vi "Controller with Indicators.vi"() -> ()   [LabVIEW 2009]
doc: "This example shows how to use Simulation Module and Control Design Toolkit together and how to transfer the controller from Design to Simulation. It also uses the 3D Picture Control Toolkit to animate the system.\nThis example is derived from the Quanser (www.quanser.com) 3 DOF Helicopter academic experiment."
uses:
  <vilib>/Simulation/Scripting/Companion Diagram/SimConfigNode/SimDog.xnode
  <vilib>/Simulation/Utility/SIMX SimTime/SIMX SimTime.xnode
  <vilib>/Simulation/SignalArithmetic/SIMX Gain/SIMX Gain.xnode
  <vilib>/Simulation/Implementation/XNodeFramework/AbstractNodes/SimX_SubsystemNode/SimX_SubsystemNode.xnode
  <vilib>/Simulation/Utility/SIMX Halt/SIMX Halt.xnode
  Heli SubVIs/cdex_unwrap signal.vi
  <vilib>/Simulation/SignalArithmetic/Implementation/NILVSim Gain.llb/SIM Gain (scalar).vi
  <vilib>/Simulation/Implementation/Shared/SIMSCR Execution Mode.ctl
  <vilib>/Simulation/Scripting/Companion Diagram/SimConfigNode/_simSolvers.ctl
  <vilib>/Simulation/Scripting/Companion Diagram/SimConfigNode/SimParams.ctl
  <vilib>/Simulation/Utility/Implementation/SIM Time.vi
  <vilib>/Simulation/Utility/Implementation/SIM Halt.vi
  NiRioSrv.dll
  <vilib>/Utility/error.llb/Error Cluster From Error Code.vi
  <vilib>/rvi/errors/niLvFpgaWhatHappensToTopLevelVI.ctl
  <vilib>/rvi/interface/common/niFpgaNodeNameForErrorReporting.ctl
  <vilib>/rvi/errors/niLvFpgaAdjustHostInterfaceError.vi
  <vilib>/rvi/interface/nirviReadWriteControl/nirviReadWriteControl.xnode
  FPGA Bitfiles/sbRIOController.lv~4B_sbRIO-9631_FPGA Main.vi.lvbitx
  <vilib>/userDefined/High Color/nirio_resource_hc.ctl
  <vilib>/rvi/interface/nirviOpenFPGA/nirviOpenFPGA.xnode
  RT/Set to PWM.vi
  <vilib>/rvi/interface/nirviCloseFPGA/nirviCloseFPGA.xnode
  Heli SubVIs/cdex_Position PID.vi
  Heli SubVIs/cdex_Elevation PID.vi
  Heli SubVIs/cdex_Pitch PID.vi
  FPGA/FPGA Main.vi
  RT/Read Encoder Data.vi
  RT/MyGlobal.vi
  <vilib>/Simulation/Implementation/Shared/SIM Bundle Sim Info.vi
  <vilib>/Simulation/Implementation/Shared/SIM Unbundle Sim Info.vi
  <vilib>/Platform/TimedLoop/XDataNode/wakeup.ctl
  <vilib>/Platform/TimedLoop/XDataNode/XDNodeRunTimeDep.lvlib
  <vilib>/Platform/TimedLoop/XDataNode/nitl_modes.ctl
  <vilib>/Platform/TimedLoop/XDataNode/timing_clust.ctl
  <vilib>/Platform/TimedLoop/XDataNode/XDataNode.xnode
  <vilib>/Simulation/Implementation/Shared/NILVSim_Initialize.vi
  <vilib>/Simulation/Implementation/Shared/NILVSim_FinishedLate.vi
  <vilib>/Simulation/Implementation/Shared/NILVSim_Manager.vi
  <vilib>/Simulation/Implementation/Shared/NILVSim_FinalizeModel.vi
  <vilib>/Simulation/Implementation/Shared/NILVSim_GetModelError.vi
  <vilib>/Platform/TimedLoop/XDataNode/loadlvalarms.vi
  <vilib>/Simulation/Implementation/Shared/SIM Fire Discrete SubVI.vi
  <vilib>/Simulation/Scripting/Editor Utilities/SIM subVI execution type.ctl
  <vilib>/Simulation/Scripting/Editor Utilities/SIM subVI tag data.ctl
  <vilib>/FPGAPlugInAG/sbRIO-9631/nirviIntfOpen_sbRIO-9631.vi
  FPGA/FPGA Main NoStartEnc.vi
  FPGA Bitfiles/sbRIOController.lv~4B_sbRIO-9631_FPGA Main NoStartE~C3.lvbitx
  <vilib>/FPGAPlugInAG/sbRIO-9631/nirviIntfClose_sbRIO-9631.vi
panel:
  in  "stop":bool
  out "error out":errorcluster
  in  "GO":bool
  in  "Clock Divider (ticks)":u16=1
  in  "PWM Period (ticks)":u32=100000
  out "Simulation Time":dbl=55.800000000000004 format="%<%H:%M:%S%1u>t"
  out "Measured Pitch Angle":dbl=0.00018032364824244914
  out "Measure Angle":dbl=14.22166948358761
  out "Measured Elevation":dbl=14.497088945408226
  in  "Position Angle Setpoint":dbl(knob) scale=-180.0..180.0
  in  "Elevation Setpoint":dbl(slide) scale=0.0..20.0 scale format="%.2f"
  out "Control Effort [Vf,Vb]":cluster{dbl, dbl}(graph)={-0.0027402268665562613, -0.002740193984032141}
  out "Travel Angle":cluster{"travel position":dbl, "signal out":dbl}(graph)={"travel position"=14.222946670967534, "signal out"=14.22166948358761}
  out "Elevation Angle":cluster{"elevation":dbl, "signal out":dbl}(graph)={"elevation"=14.285714285714286, "signal out"=14.497088945408226}
  # "X"
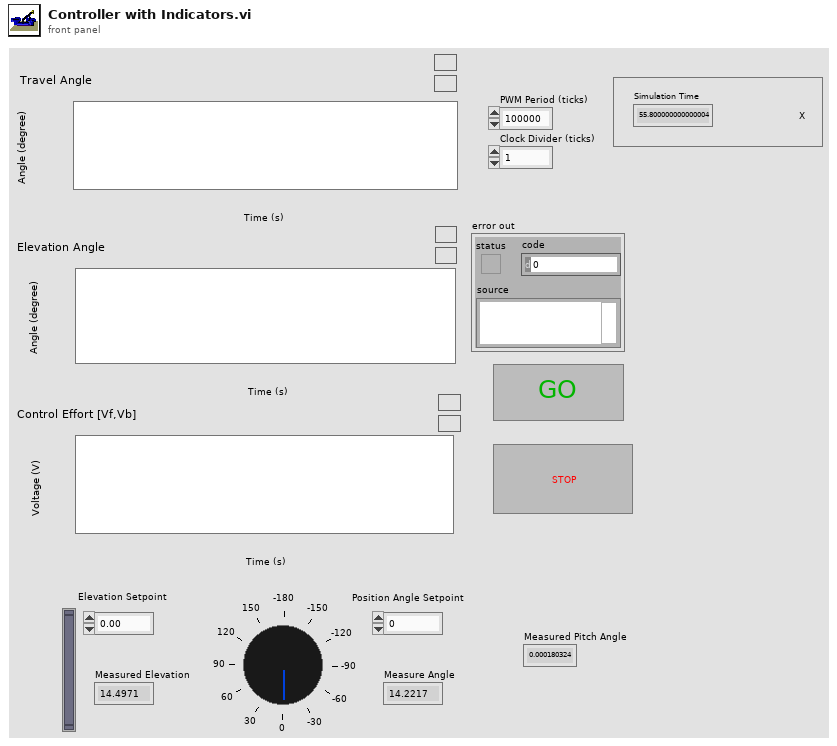
[diagram p1: front panel]
types:
  T1 = cluster{"travel position":dbl, "signal out":dbl}[]
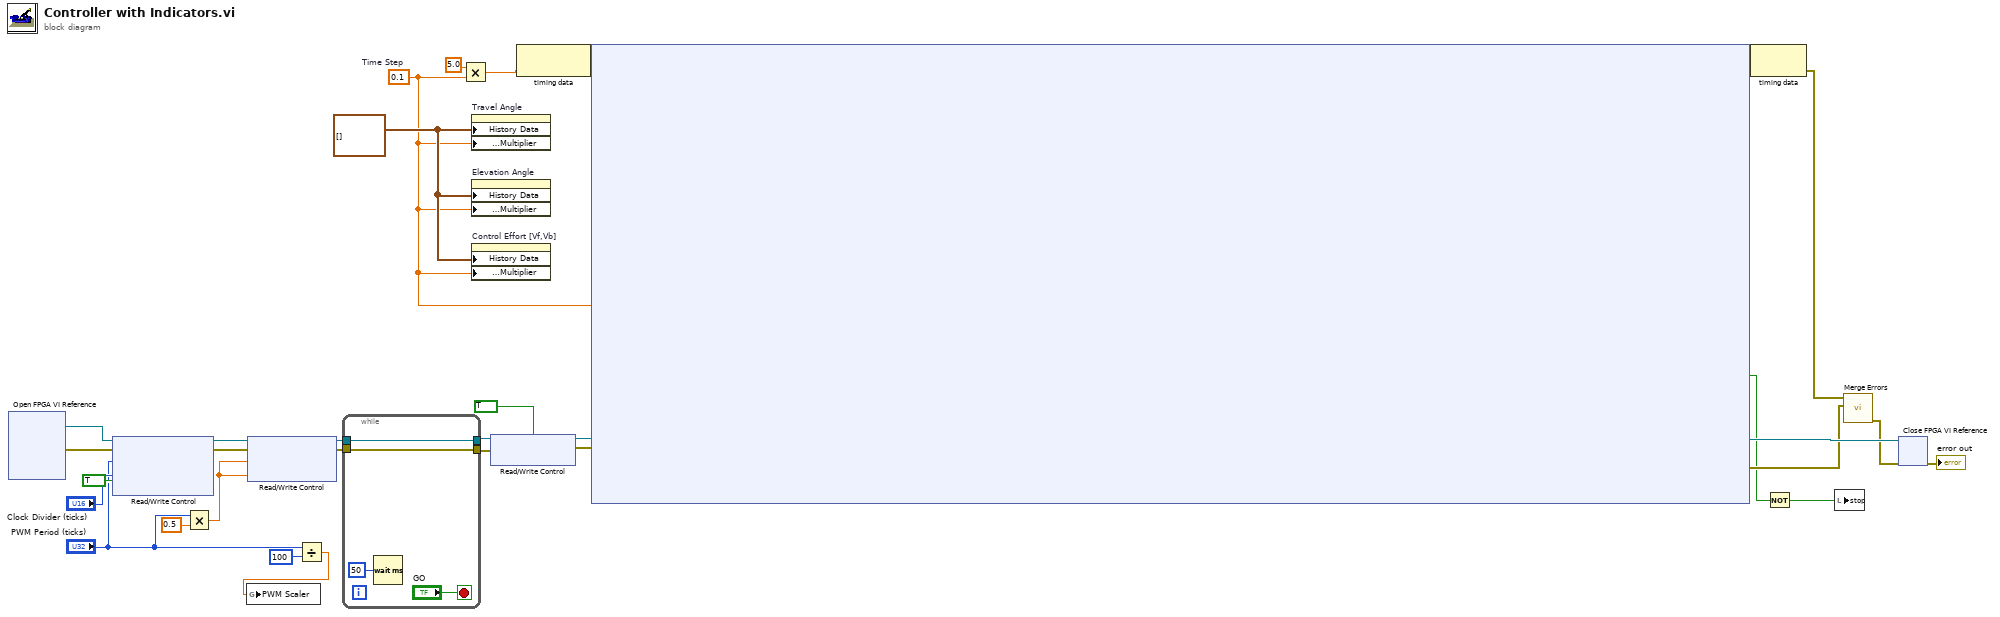
[diagram p0: block diagram]
diagram:
  w26 = 0.1  # Time Step
  w31 = T1 [] ("History Data")
  n1 = xnode "Open FPGA VI Reference"() -> ("FPGA VI Reference Out"=w22:refnum<k20>, "error out"=w23:errorcluster)  [unwired: 2 in]
  n2 = xnode "Read/Write Control"("FPGA VI Reference In"=w22, "error in"=w23, "PWM Period (ticks)"="PWM Period (ticks)", "Clock Divider"="Clock Divider (ticks)", "ENC In Clock"=TRUE) -> ("FPGA VI Reference Out"=w9:refnum<k20>, "error out"=w10:errorcluster)
  n3 = Multiply(x="PWM Period (ticks)", y=sgl 0.5) -> (x*y=w13:sgl)
  n4 = xnode "Read/Write Control"("FPGA VI Reference In"=w9, "error in"=w10, "Fan High Time 1"=w13, "Fan High Time 2"=w13) -> ("FPGA VI Reference Out"=w7:refnum<k20>, "error out"=w8:errorcluster)
  n5 = Divide(x="PWM Period (ticks)", y=u32 100) -> (x/y=w1:dbl)
  n6 = global write "MyGlobal.vi" "PWM Scaler"(w1) -> ()
  n7 = while {
    tunnel: w8 -> [w32]
    tunnel: w7 -> [w33]
    tunnel: [w33] -> w5
    tunnel: [w32] -> w6
    stop <- "GO" stop-if-true
    n8 = Wait (ms)(milliseconds to wait=u32 50) -> ()  [unwired: 1 out]
  }
  n9 = Multiply(x=5.0 ("y"), y=w26) -> (x*y=w28:dbl)
  n10 = property on="Travel Angle" class="WaveformChart (strict)"("History Data"=w31, "X Scale.Offset and Multiplier:Multiplier"=w26) -> ()  [unwired: 2 in, 2 out]
  n11 = property on="Elevation Angle" class="WaveformChart (strict)"("History Data"=w31, "X Scale.Offset and Multiplier:Multiplier"=w26) -> ()  [unwired: 2 in, 2 out]
  n12 = property on="Control Effort [Vf,Vb]" class="WaveformChart (strict)"("History Data"=w31, "X Scale.Offset and Multiplier:Multiplier"=w26) -> ()  [unwired: 2 in, 2 out]
  n13 = xnode "Read/Write Control"("FPGA VI Reference In"=w5, "error in"=w6, "Start Encoders"=TRUE) -> ("FPGA VI Reference Out"=w2:refnum<k20>, "error out"=w3:errorcluster)
  n14 = node-c288(w28) -> (w30:variant)
  n15 = node-c254 ("Simulation Loop")(w26, w30, w3, w2) -> (w29:variant, w17:errorcluster, w20:refnum<k20>, w12:bool)
  n16 = node-c288(w29) -> (w18:errorcluster)
  n17 = Not(x=w12) -> (.not. x?=w11:bool)
  n18 = local write "stop"(w11) -> ()
  n19 = call <vilib>:"Merge Errors.vi"("error in 2 (no error)"=w17, "error in 1 (no error)"=w18) -> ("error out"=w16:errorcluster)  [unwired: 5 in]
  n20 = xnode "Close FPGA VI Reference"("FPGA VI Reference In"=w20, "error in"=w16) -> ("error out"=→"error out":errorcluster)
